vi "Format UI Size.vi"() -> (0 "error out":errorcluster)   [LabVIEW 2019, in "Configuration Tool.lvlib"]
uses:
  Configuration Tool.lvlib
  <vilib>/Utility/miscctls.llb/LVPositionTypeDef.ctl
  <vilib>/Utility/miscctls.llb/LVBoundsTypeDef.ctl
  <vilib>/Utility/miscctls.llb/LVPointTypeDef.ctl
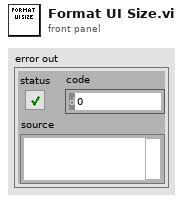
[diagram p1: front panel]
types:
  T1 = typedef "LVPointTypeDef.ctl" = cluster{"Horizontal":i16, "Vertical":i16}
  T2 = typedef "LVBoundsTypeDef.ctl" = cluster{"Width":u32, "Height":u32}
  T3 = typedef "LVPositionTypeDef.ctl" = cluster{"Left":i32, "Top":i32}
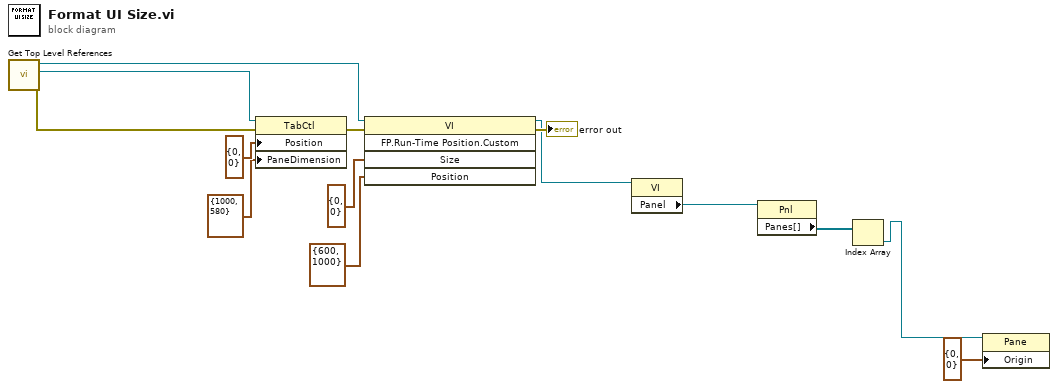
[diagram p0: block diagram]
diagram:
  n1 = call "Get Top Level References.vi"() -> ("error out"=w9:errorcluster, "Main UI Tab Ref"=w7:refnum<vi>, "VI ref"=w8:refnum<vi>)  [unwired: 9 in]
  n2 = property on="Property Node" class="TabCtl"(reference=w7, error in=w9, "Position"=T3 {"Left"=0, "Top"=0}, "PaneDimension"=T2 {"Width"=1000, "Height"=580} ("Tab Control Pane Dimension")) -> (error out=w13:errorcluster)  [unwired: 1 out]
  n3 = invoke class="VI" method="FP.Run-Time Position.Custom"(reference=w8, error in=w13, "Size"=cluster{"Top":i16, "Left":i16} {"Top"=0, "Left"=0} ("Position"), "Position"=cluster{"Height":i16, "Width":i16} {"Height"=600, "Width"=1000} ("Size")) -> (reference out=w5:refnum<vi>, error out=→"error out":errorcluster)  [unwired: 1 in, 3 out]
  n4 = property on="Property Node" class="VI"(reference=w5) -> ("Panel"=w4:refnum<vi>)  [unwired: 1 in, 2 out]
  n5 = property on="Property Node" class="Pnl"(reference=w4) -> ("Panes[]"=w3:refnum<vi>[])  [unwired: 1 in, 2 out]
  n6 = Index Array(array=w3) -> (element=w2:refnum<vi>)  [unwired: 1 in]
  n7 = property on="Property Node" class="Pane"(reference=w2, "Origin"=T1 {"Horizontal"=0, "Vertical"=0}) -> ()  [unwired: 1 in, 2 out]
